vi "String To Array.vi"(5 "Unescape? [F]":bool, 7 "Strip Whitespace? [T]":bool=TRUE, 8 "error in (no error)":errorcluster, 10 "resulting string":string, 11 "Registry Object":refnum<class "Carya Config.lvclass">) -> (0 "error out":errorcluster, 2 "Array":string[](array[string]), 3 "Registry Object":refnum<class "Carya Config.lvclass">)   [LabVIEW 2013, in "Carya Config.lvclass"]
doc: "Copyright 2018, Carya Automatisering, Wiebe Walstra."
uses:
  Carya Config.lvclass
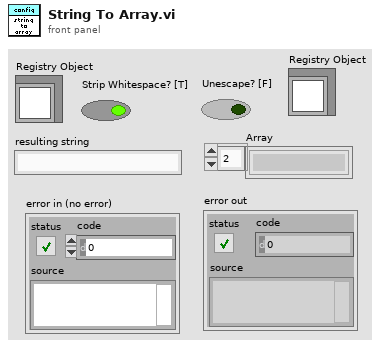
[diagram p1: front panel]
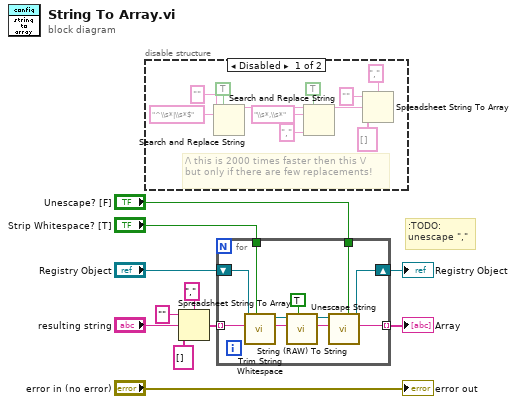
[diagram p0: block diagram]
diagram:
  # ":TODO:\nunescape \",\""
  n1 = disable-structure shown="Disabled" {
    frame Disabled {
      # "/\\ this is 2000 times faster then this \\/\nbut only if there are few replacements!"
      n2 = Search and Replace String(replace all?=TRUE ("replace all? (F)"), input string="", search string="^\\s*|\\s*$") -> (result string=w17:string)  [unwired: 5 in, 3 out]
      n3 = Search and Replace String(replace all?=TRUE ("replace all? (F)"), input string=w17, search string="\\s*,\\s*", replace string="," ("replace string (\"\")")) -> (result string=w12:string)  [unwired: 4 in, 3 out]
      n4 = Spreadsheet String To Array(delimiter (Tab)=",", format string="", spreadsheet string=w12, array type (2D Dbl)=string[] []) -> ()  [unwired: 1 out]
    }
    frame Enabled {
    }
  }
  n5 = Spreadsheet String To Array(delimiter (Tab)=",", format string="", spreadsheet string="resulting string", array type (2D Dbl)=string[] []) -> (array=w5:string[])
  n6 = for {
    tunnel: w5 -> [w33] mode=indexing
    tunnel: [w30] -> w9 mode=indexing
    shift-right: [w31] -> w3
    shift-left: "Registry Object" -> [w32]
    tunnel: "Strip Whitespace? [T]" -> [w29]
    tunnel: "Unescape? [F]" -> [w28]
    n7 = call-dynamic "Trim String Whitespace.vi"("Strip Whitespace? [T]"=w29, "String"=w33, "Registry Object"=w32) -> ("Trimmed string"=w25:string, "Registry Object"=w27:refnum<class "Carya Config.lvclass">)  [unwired: 6 in, 1 out]
    n8 = call-dynamic "String (RAW) To String.vi"("Raw String to String? [T]"=TRUE, "String (RAW)"=w25, "Registry Object"=w27) -> ("String"=w24:string, "Registry Object"=w26:refnum<class "Carya Config.lvclass">)  [unwired: 6 in, 1 out]
    n9 = call-dynamic "Unescape String.vi"("Unescape? [T]"=w28, "String"=w24, "Registry Object"=w26) -> ("Unescaped string"=w30:string, "Registry Object"=w31:refnum<class "Carya Config.lvclass">)  [unwired: 6 in, 1 out]
  }
  "Registry Object" <- w3
  "Array" <- w9
  "error out" <- "error in (no error)"
